vi "Welcome window.vi"(11 "error in (no error)":errorcluster) -> (8 "OK":bool, 10 "Quick start":bool, 15 "error out":errorcluster)   [LabVIEW 2011]
doc: "Welcome screen, with basic options"
uses:
  Tool/Tool selectro.ctl
  Tool/Stroker selectro.ctl
  Tool/Driller selectro.ctl
  Tool/Tractor selectro.ctl
  Project control/Project infor with project path.ctl
  Project control/Project in icluster.ctl
  Job setup/Job and site cluster.ctl
  emi cndiates/List of all contrys(combo box).ctl
  Job setup/Tool registration ID.ctl
  Project control/Run Information.ctl
  Tool/List of tools.ctl
  <vilib>/Utility/libraryn.llb/Check if File or Folder Exists.vi
  emi Lib/Basic/0 - General/App/Version/Private/_emi_Version Holder.vi
  <vilib>/Platform/browser.llb/Open URL in Default Browser (path).vi
  <vilib>/Platform/browser.llb/Open URL in Default Browser (string).vi
panel:
  in  "Tool selector":T1
  out "Project name":string
  in  "Quick start":bool
  in  "Sequenze":bool
  out "User name":string="TEST"
  in  "Change User":bool
  in  "Tool Builder":bool
  in  "IO Setup":bool
  in  "Data Sheets":bool
  in  "Promo":bool
  out "Version Full":string="Version"
  in  "Web Qinterra":bool
  in  "Web Mar-In":bool
  in  "Help":bool
  in  "Cancel":bool
  in  "OK btn":bool
  # "Beagle"
  # "Welcome"
  # "Please select operation mode to the right, then press Continue. \nFor more information press F1"
  # "Current project:"
  # "Tab header s can be changed as wanted\n\nCustom can be used for completly ccutom behavior,\nmust then highjack  an other hidden page, for settings"
  # "Add custom behavior taht cvan not be replicated by a simple cluster with valisdity checking"
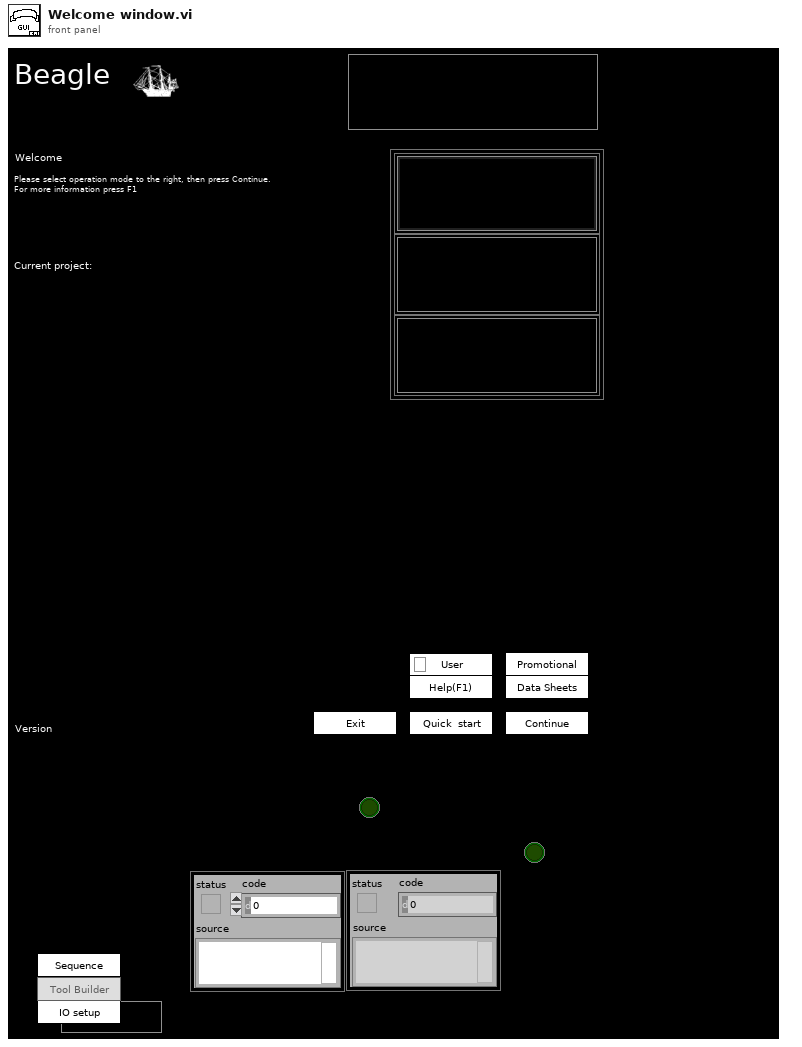
[diagram p1: front panel]
types:
  T1 = typedef "Tool selectro.ctl" = enum32{"Radio Selection 1", "Radio Selection 2", "Radio Selection 3"}
  T2 = enum32{"Invalid", "Default", "Floating", "Floating/Auto-Hide", "Modal"}
  T3 = enum16{"GET", "SET", "Get from Ini", "Put in Ini"}
  T4 = typedef "User Indikator.ctl" = cluster{"User Name":string, "Super User":T5}
  T5 = typedef "Super User bool indikator.ctl" = bool
  T6 = typedef "Options  All pages and custom.ctl" = cluster{"P 1 (App)":T7, "P 2":T8, "P 3":T9, "P 4":T12, "P 5":T17, "P 6 (Err)":T18, "P 7 (Expert)":T19, "P 8 (Depth)":T21, "C 1":T22, "C 2":T23}
  T7 = typedef "Options Page 1 (App).ctl" = cluster{"Result files":path, "PCP Interface":string, "Tractor/Stroker Interface":string, "Tractor Interface":string, "Modem Status Interface":string, "Audible Alarm":bool, "Force alarm on Technical":bool, "Force alarm on HH":bool, "Force alarm on LL":bool, "Force alarm on H":bool, "Force alarm on L":bool}
  T8 = typedef "Options Page 2.ctl" = cluster{"Solenoid & Relay latching time":u16, "Tractor relay 1":dbl, "Tractor relay 2":dbl, "Tractor Solenoid limit":dbl}
  T9 = typedef "Options Page 3.ctl" = cluster{"Min resistance":dbl, "Max resistance":dbl, "Head voltage range":T10, "Max voltage jump":dbl, "Maximum resistance change":dbl, "Start Telemetry Voltage":dbl, "Start Telemetry Timeout":dbl, "Start Motor Voltage":dbl, "Stop Motor Voltage":dbl, "Pass Mode Warning Voltage":dbl, "Relay Switch Voltage":dbl, "Relay Status Loss Voltage":dbl, "Samples to average":i32, "PSU type DO NOT USE":T11, "Magna OVP":dbl, "Magna Current Limit":dbl}
  T10 = typedef "PCP type List.ctl" = enum16{"0 - 350V", "0 - 450V", "0 - 600V"}
  T11 = typedef "PSU Type.ctl" = enum16{"Unipower", "Magna 8.3A", "Magna 12A", "None"}
  T12 = typedef "Options Page 4.ctl" = cluster{"Solenoid & Relay latching time":u16, "Stroker relay 1":dbl, "Stroker Relay 2":dbl, "Stroker Solenoid limit":dbl, "Force det.":T13, "Stroke force lim.":dbl, "Anchor Enabled Pressure":dbl, "Tacometer puls":dbl, "Default anchor behavior":T14, "Default stroker behavior":T15, "Default stroker force limit (tonne)":dbl, "Slips Size":T16}
  T13 = typedef "Stroke force selector.ctl" = enum16{"Stroke in = node 1", "Strok out = node 1"}
  T14 = typedef "Default anchor behavior.ctl" = enum16{"Do nothing", "Set Anchor", "Release Anchor"}
  T15 = typedef "Default stroker behavior.ctl" = enum16{"Do nothing", "Stop", "Go Out", "Go In"}
  T16 = typedef "Slips Type Radio.ctl" = enum32{"No Selection", "338 MRS", "3,9 MRS"}
  T17 = typedef "Options Page 5.ctl" = cluster{"Solenoid & Relay latching time":u16, "Driller relay 1":dbl, "Driller Relay 2":dbl, "Driller  Solenoid limit":dbl}
  T18 = typedef "Options Page 6 (Err).ctl" = cluster{"Error and event files":path}
  T19 = typedef "Options Page 7 (Expert).ctl" = cluster{"Show Debug":bool, "Log debug messages":bool, "Additional debug messages":bool, "Start Beagle with Simulator data":bool, "Workshop mode":bool, "Modem baud":u16, "enumCANCOM":bool, "Modem sim":T20, "Telemetry Timeout Disable":i32, "Buffer size":i32, "Upd regular data":bool, "Cable comp":cluster{"VMOD1 Voltage(V)":dbl, "VMOD2 Voltage(V)":dbl}}
  T20 = typedef "Modem simulation setup.ctl" = cluster{"Modem dealay sim":bool, "Sim baud Tx":u16, "Bit Error fraction Tx":dbl, "Sim baud Rx":u16, "Bit Error fraction Rx":dbl}
  T21 = typedef "Options Page 8 (Depth).ctl" = cluster{"Winch Spool Circumference":dbl, "Winch Pulses per Revolution":dbl, "Current Depth":dbl}
  T22 = typedef "Options Custom 1.ctl" = cluster{"Depth Updated":bool, "Depth Offset":dbl}
  T23 = typedef "Options Custom 2.ctl" = cluster{"Placeholder":bool}
  T24 = typedef "Project infor with project path.ctl" = cluster{"Project path":path, "data":T25, "Comment":string}
  T25 = typedef "Project in icluster.ctl" = cluster{"Job and Site":T26, "Tool":T28, "Run Information":T29}
  T26 = typedef "Job and site cluster.ctl" = cluster{"Project Number":string, "Client Company":string, "Country":T27, "Field":string, "Rig":string, "Well":string}
  T27 = typedef "List of all contrys(combo box).ctl" = string
  T28 = typedef "Tool registration ID.ctl" = cluster{"Tractor type":string, "Tool":string, "Serial #":string}
  T29 = typedef "Run Information.ctl" = cluster{"Active Run":bool, "String Check Rec":bool, "Run Number":i32, "Time of File Start":string}
  T30 = enum8{"Enabled", "Disabled", "Disabled and Grayed Out"}
  T31 = typedef "emi_Version Info.ctl" = cluster{"Name":string, "Major":i16, "Minor":i16, "Fix":i16, "Build":i32, "Type":enum16{"Alfa", "Beta", "Stable"}, "Dev":bool, "Version Name":string, "Date":timestamp}
  T32 = typedef "List of tools.ctl" = enum16{"Stroker", "Driller", "Tractor"}
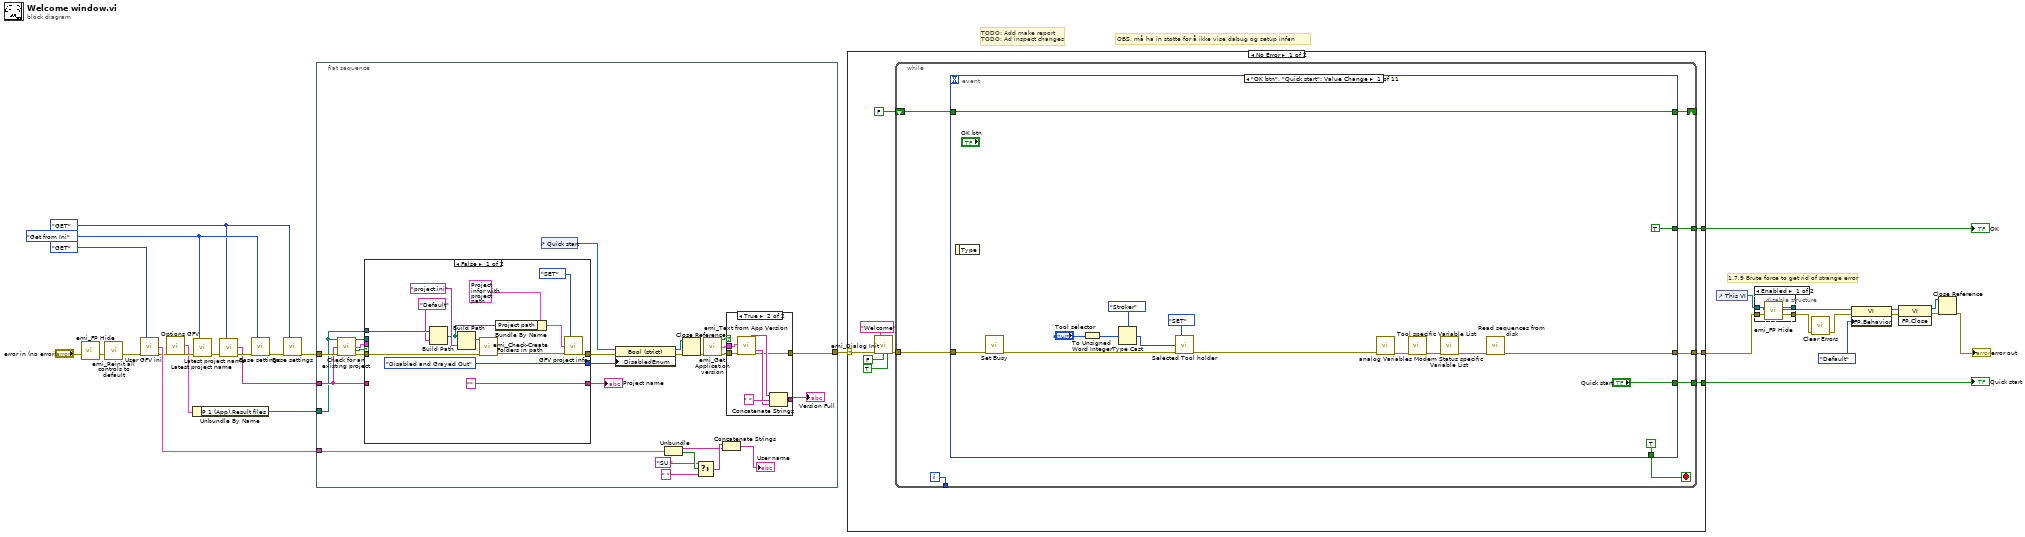
[diagram p0: block diagram]
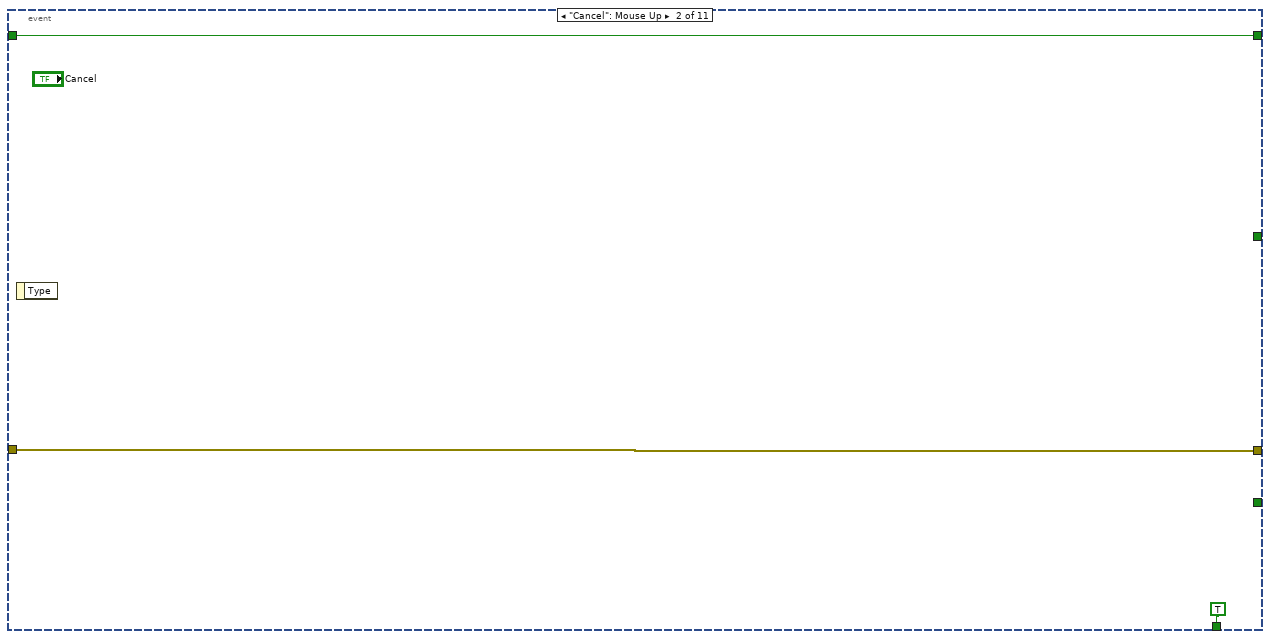
[diagram p3: hidden frame]
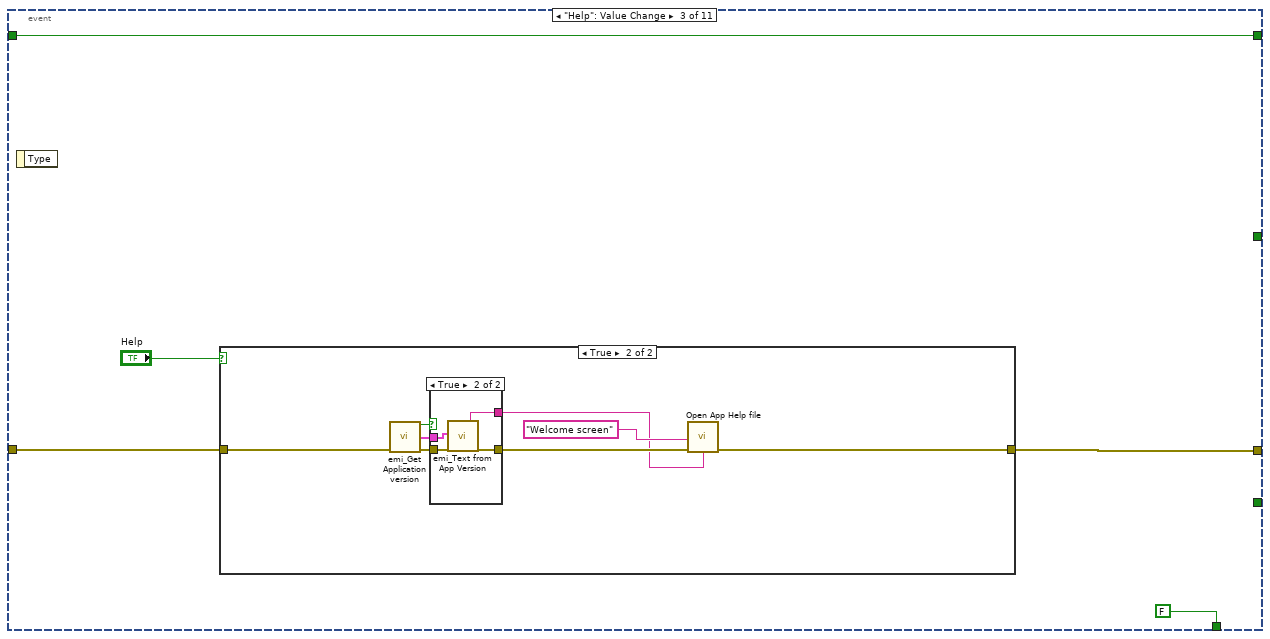
[diagram p4: hidden frame]
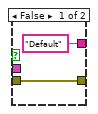
[diagram p6: hidden frame]
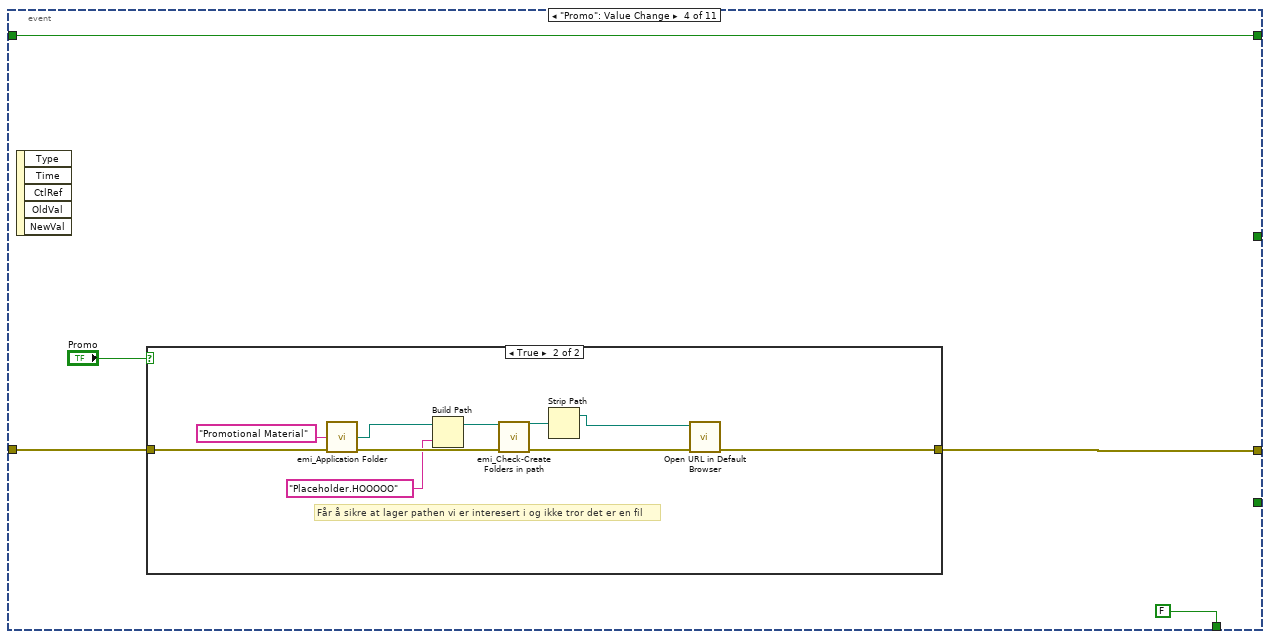
[diagram p7: hidden frame]
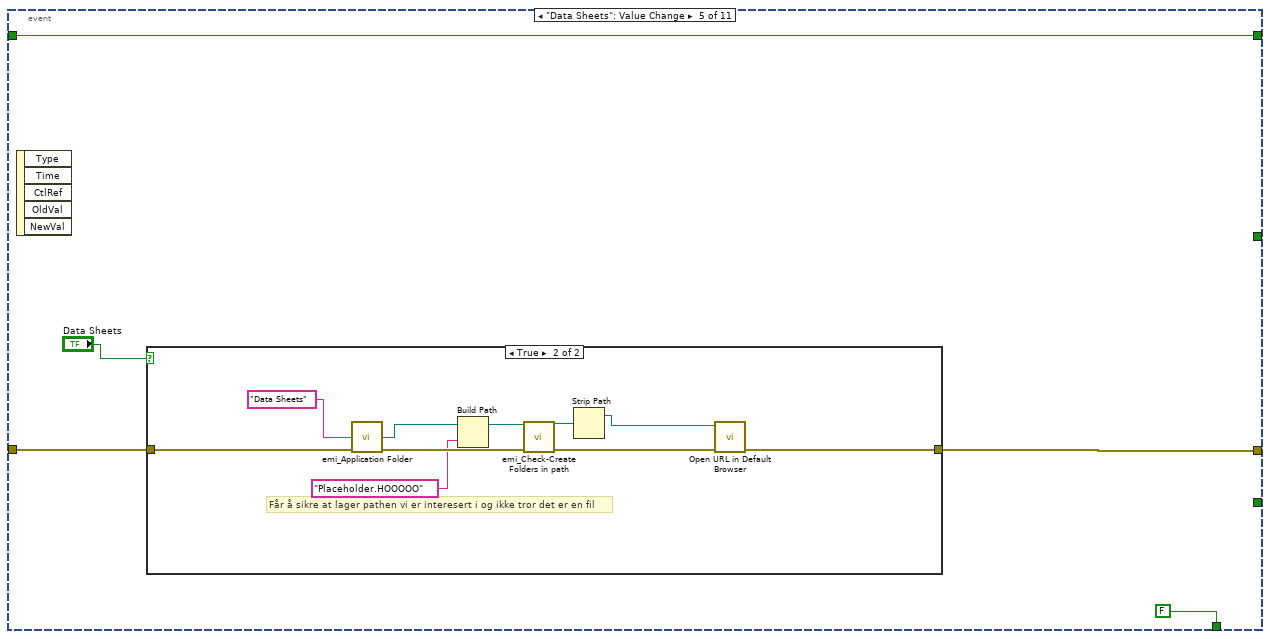
[diagram p9: hidden frame]
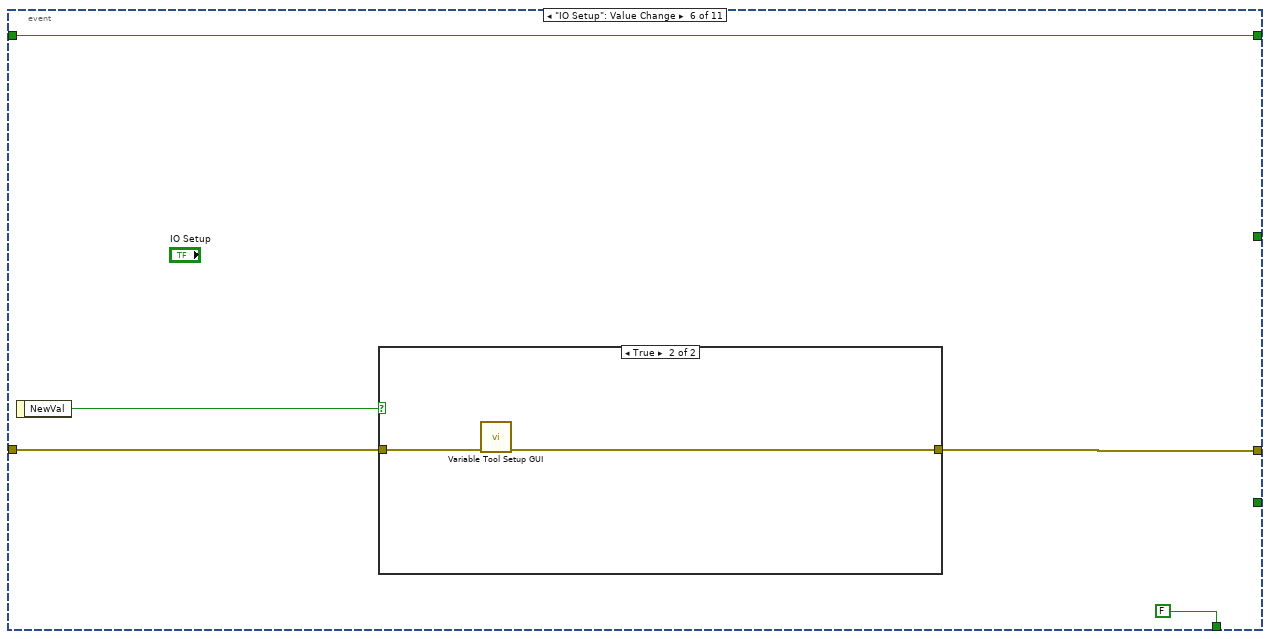
[diagram p11: hidden frame]
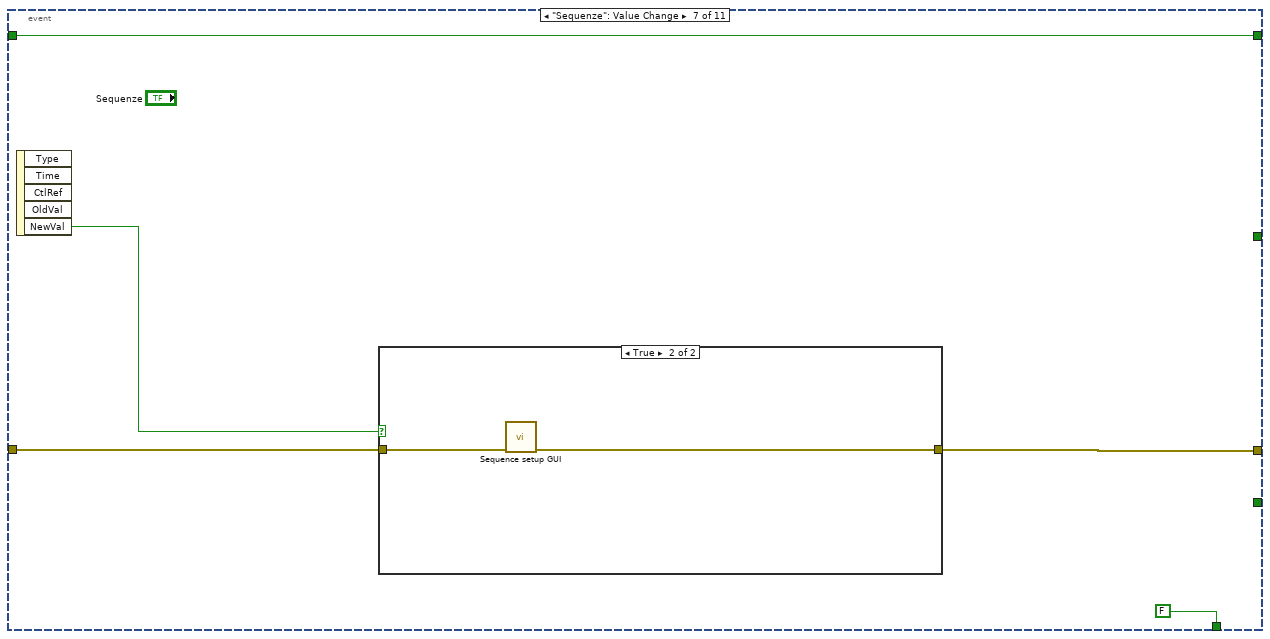
[diagram p13: hidden frame]
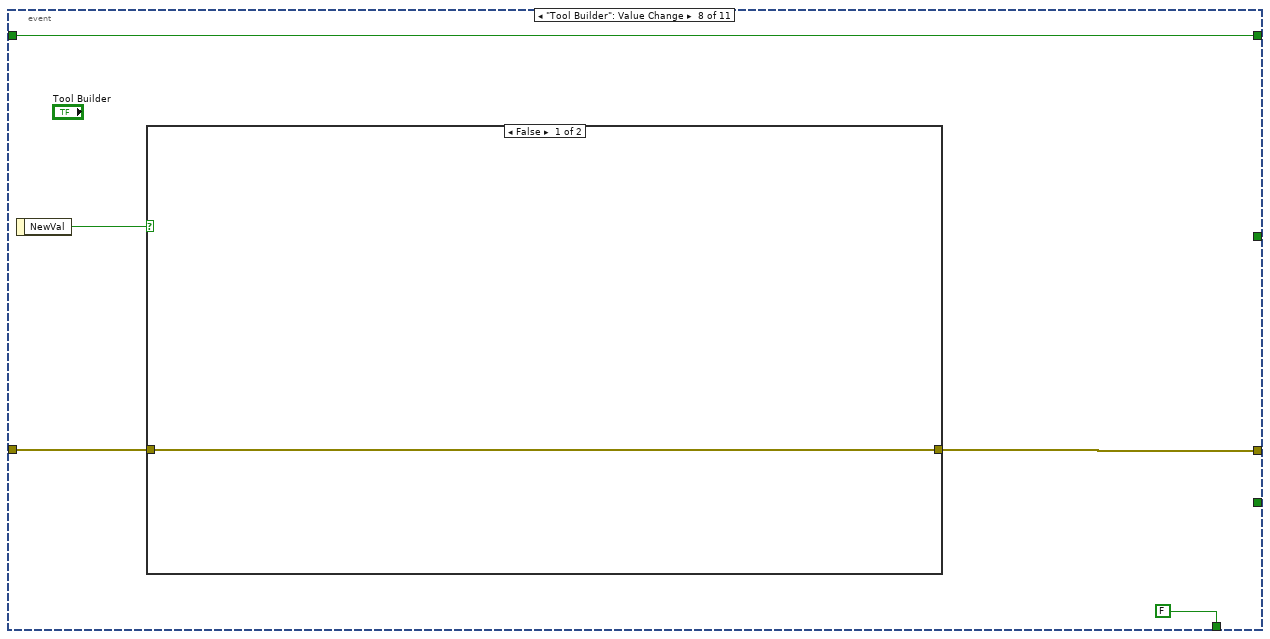
[diagram p15: hidden frame]
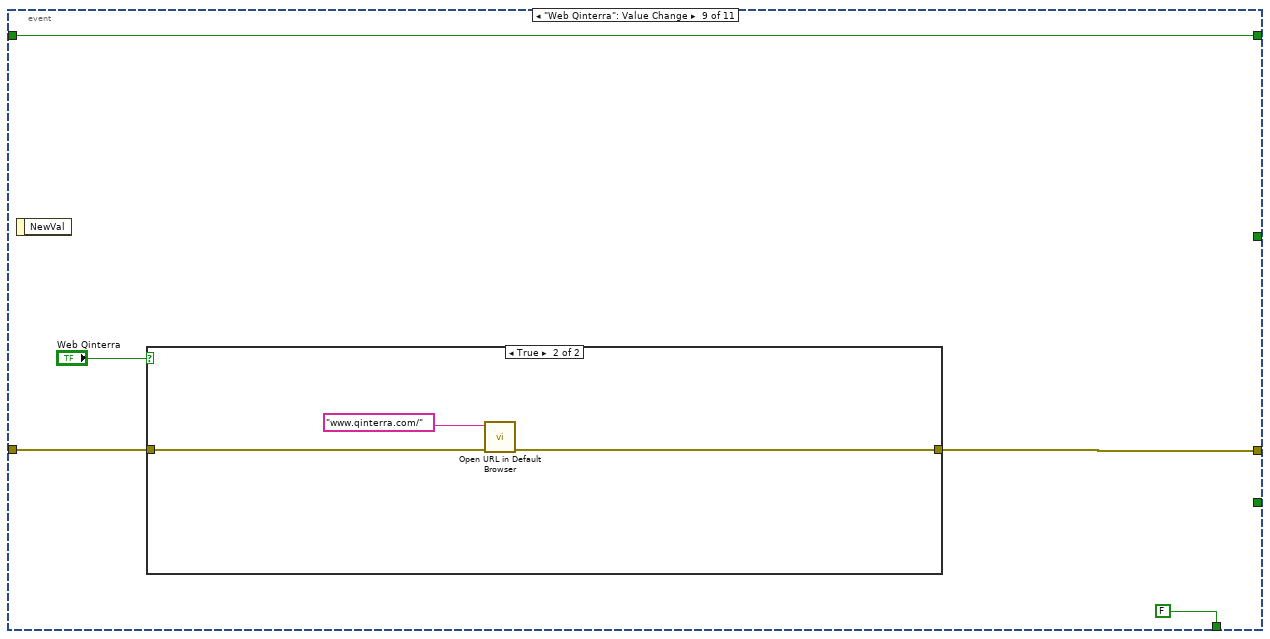
[diagram p17: hidden frame]
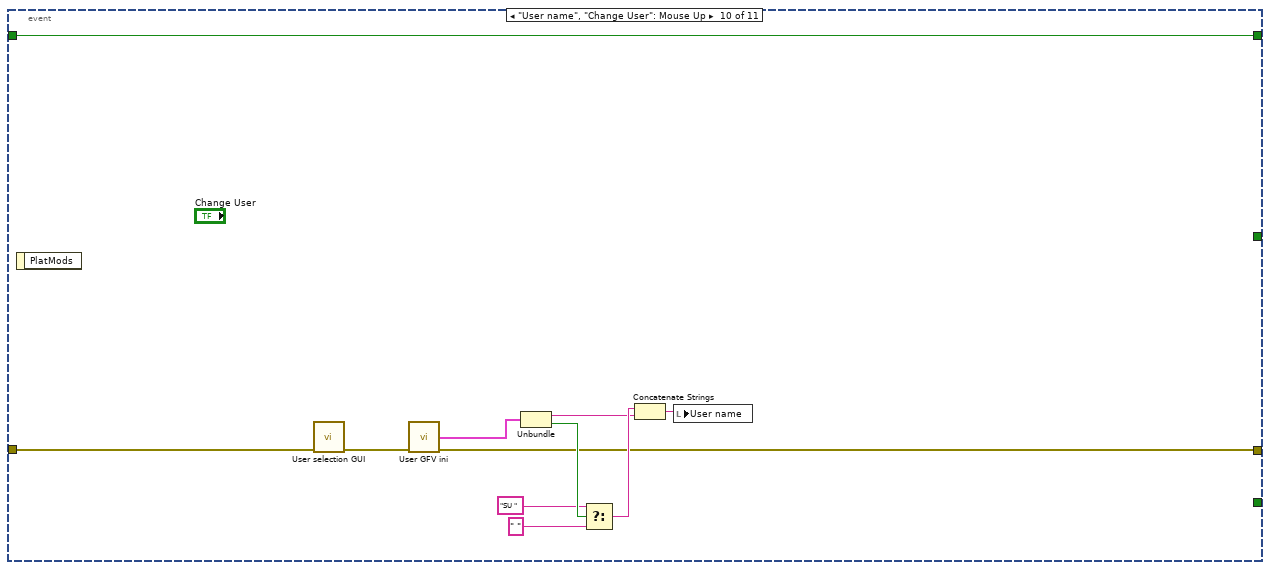
[diagram p19: hidden frame]
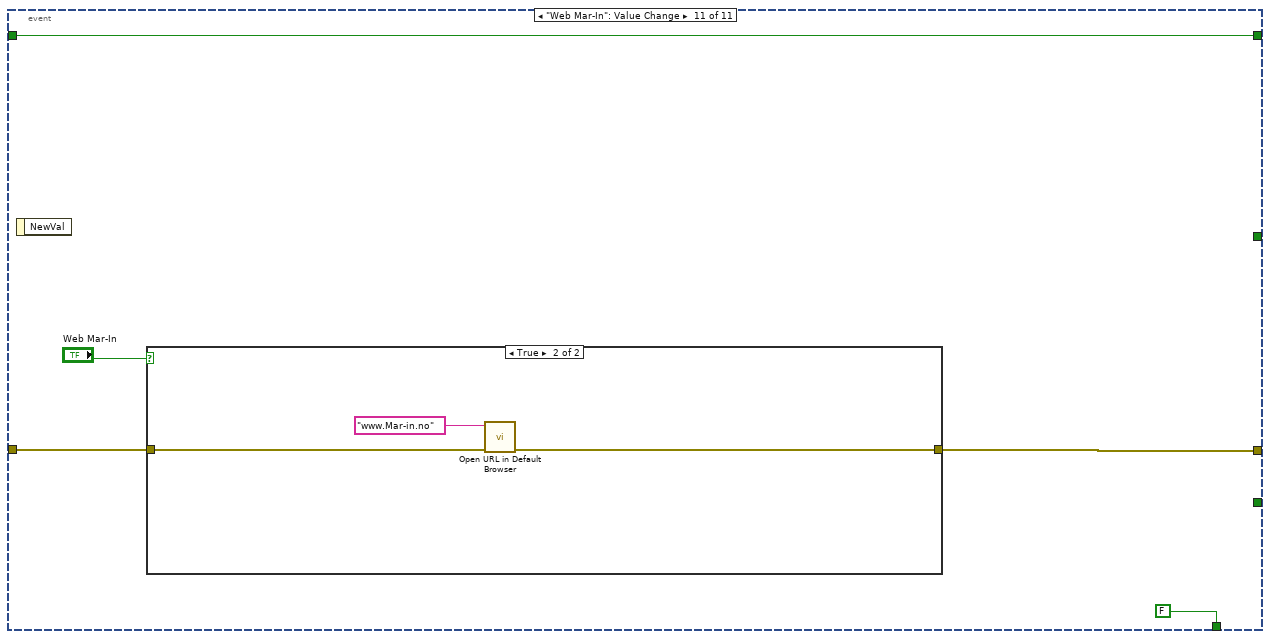
[diagram p20: hidden frame]
diagram:
  w16 = T3."GET" ("Action(GET)")
  w17 = T3."Get from Ini" ("Action(GET)")
  # "1.7.9 Brute force to get rid of strange error"
  # "OBS, må ha in støtte for å ikke vise dabug og setup infen"
  # "TODO: Add make report\nTODO: Ad inspect changes"
  n1 = call "emi_FP Hide.vi"("error in (no error)"="error in (no error)") -> ("error out"=w26:errorcluster)  [unwired: 13 in, 1 out]
  n2 = call "emi_Reinit all controls to default.vi"("error in (no error)"=w26) -> ("error out"=w1:errorcluster)  [unwired: 13 in, 1 out]
  n3 = call "User GFV ini.vi"("Action(GET)"=T3."GET", "error in (no error)"=w1) -> ("User ID out"=w23:T4, "error out"=w14:errorcluster)  [unwired: 12 in]
  n4 = call "Options GFV.vi"("error in (no error)"=w14) -> ("Options"=w12:T6, "error out"=w13:errorcluster)  [unwired: 16 in, 1 out]
  n5 = Unbundle By Name(w12) -> ("P 1 (App).Result files"=w11:path)
  n6 = call "Latest project name.vi"("Action(GET)"=w17, "error in (no error)"=w13) -> ("error out"=w19:errorcluster)  [unwired: 12 in, 1 out]
  n7 = call "Latest project name.vi"("Action(GET)"=w16, "error in (no error)"=w19) -> ("Project name out"=w15:string, "error out"=w18:errorcluster)  [unwired: 12 in]
  n8 = call "Base settings.vi"("Action(GET)"=w17, "error in (no error)"=w18) -> ("error out"=w22:errorcluster)  [unwired: 12 in, 1 out]
  n9 = call "Base settings.vi"("Action(GET)"=w16, "error in (no error)"=w22) -> ("error out"=w21:errorcluster)  [unwired: 12 in, 1 out]
  n10 = flat-sequence {
    tunnel: [w52] -> w25
    tunnel: w21 -> [w45]
    tunnel: w23 -> [w31]
    tunnel: w15 -> [w42]
    tunnel: w11 -> [w32]
    frame #0 {
      n11 = call "Check for an existing project.vi"("Base folder"=w32, "Project name"=w42, "error in"=w45) -> ("Project folder"=w34:path, "data"=w33:T25, "Project exists"=w43:bool, "error out"=w44:errorcluster)  [unwired: 5 in, 4 out]
      n12 = case shown="False" w43 {
        tunnel: [w60 w74] -> w39
        tunnel: w44 -> [w64 w75]
        tunnel: w42 -> [_ w71]
        tunnel: ["" ("f") w71] -> w41
        tunnel: [T30."Disabled and Grayed Out" ("Disabled") T30."Enabled" ("Disabled")] -> w35
        tunnel: w34 -> [_ w76]
        tunnel: w33 -> [_ w70]
        tunnel: w32 -> [w67 _]
        frame False {
          n13 = Build Path(base path=w67, name or relative path="Default") -> (appended path=w57:path)
          n14 = Build Path(base path=w57, name or relative path="project.ini") -> (appended path=w63:path)
          n15 = call "emi_Check-Create Folders in path.vi"("Path including file"=w63, "error in (no error)"=w64) -> ("error out"=w59:errorcluster)  [unwired: 11 in, 2 out]
          n16 = Bundle By Name(cluster=T24 {"Project path"=path "", "data"={"Job and Site"={"Project Number"="Default", "Client Company"="", "Country"="", "Field"="", "Rig"="", "Well"=""}, "Tool"={"Tractor type"="", "Tool"="", "Serial #"=""}, "Run Information"={"Active Run"=FALSE, "String Check Rec"=FALSE, "Run Number"=0, "Time of File Start"=""}}, "Comment"=""} ("Project info"), "Project path"=w57) -> (w61:T24)
          n17 = call "GFV project info.vi"("Action(GET)"=enum16{"GET", "SET"}."SET", "Project info in"=w61, "error in (no error)"=w59) -> ("error out"=w60:errorcluster)  [unwired: 11 in, 1 out]
        }
        frame True {
          n18 = Bundle(cluster=T24 {"Project path"=path "", "data"={"Job and Site"={"Project Number"="", "Client Company"="", "Country"="", "Field"="", "Rig"="", "Well"=""}, "Tool"={"Tractor type"="", "Tool"="", "Serial #"=""}, "Run Information"={"Active Run"=FALSE, "String Check Rec"=FALSE, "Run Number"=0, "Time of File Start"=""}}, "Comment"=""} ("Project info"), "Project path"=w76, "data"=w70) -> (w72:T24)  [unwired: 1 in]
          n19 = call "GFV project info.vi"("Action(GET)"=enum16{"GET", "SET"}."SET", "Project info in"=w72, "error in (no error)"=w75) -> ("error out"=w74:errorcluster)  [unwired: 11 in, 1 out]
        }
      }
      "Project name" <- w41
      n20 = control-ref of="Quick start"() -> (w40:refnum<vi>)
      n21 = property class="Bool (strict)"(reference=w40, error in=w39, "DisabledEnum"=w35) -> (reference out=w36:refnum<vi>, error out=w37:errorcluster)
      n22 = Unbundle(w31) -> ("User Name"=w47:string, "Super User"=w51:T5)
      n23 = Close Reference(reference=w36, error in (no error)=w37) -> (error out=w38:errorcluster)
      n24 = Select(t="SU " ("User Name"), s=w51, f=" " ("User Name")) -> (s? t:f=w48:string)
      n25 = call "emi_Get Application version.vi"("error in (no error)"=w38) -> ("Version has been set"=w56:bool, "Version Info out"=w55:T31, "error out"=w54:errorcluster)  [unwired: 12 in]
      n26 = Concatenate Strings(w48, w47) -> (→"User name":string)
      n27 = case shown="True" w56 {
        tunnel: ["" w87] -> w53
        tunnel: w54 -> [w79 w85]
        tunnel: w55 -> [_ w84]
        tunnel: [w79 w81] -> w52
        frame False {
        }
        frame True {
          n28 = call "emi_Text from App Version.vi"("Version Info"=w84, "error in (no error)"=w85) -> ("Name"=w83:string, "Full version"=w82:string, "error out"=w81:errorcluster)  [unwired: 8 in, 7 out]
          n29 = Concatenate Strings(w83, " " ("string"), w82) -> (w87:string)
        }
      }
      "Version Full" <- w53
    }
  }
  n30 = case shown="No Error" w25 {
    selector: w25 -> [w91 w233]
    tunnel: [w96 FALSE] -> w29
    tunnel: [w95 w233] -> w28
    tunnel: [w88 _] -> w20
    frame No Error {
      n31 = call "emi_Dialog Init.vi"("Header String(\"\")"="Welcome" ("Header String(\"\")"), "error in"=w91, "Set BG Color(T)"=FALSE, "Modal(T)"=TRUE) -> ("error out"=w94:errorcluster)  [unwired: 11 in]
      n32 = while {
        tunnel: [w104] -> _
        tunnel: w94 -> [w102]
        tunnel: [w101] -> w95
        tunnel: [w100] -> w96
        shift-right: [w98] -> _
        shift-left: FALSE -> [w99]
        tunnel: [w97] -> w88
        i -> [w104]
        stop <- w103 stop-if-true
        n33 = event shown="[0] \"OK btn\", \"Quick start\": Value Change" {
          selector: _ -> [_ _ _ _ _ _ _ _ _ _ _]
          dyn-events: _ -> [_ _ _ _ _ _ _ _ _ _ _]
          timeout: _ -> [_ _ _ _ _ _ _ _ _ _ _]
          tunnel: [TRUE TRUE FALSE FALSE FALSE FALSE FALSE FALSE FALSE _ FALSE] -> w103
          tunnel: w102 -> [w117 w122 w126 w146 w162 w178 w186 w194 w201 w212 w221]
          tunnel: [w115 w122 w127 w147 w163 w179 w187 w195 w202 w208 w222] -> w101
          tunnel: [TRUE _ _ _ _ _ _ _ _ _ _] -> w100
          tunnel: w99 -> [w119 w121 w124 w145 w161 w177 w185 w193 w200 w218 w220]
          tunnel: [w119 w121 w124 w145 w161 w177 w185 w193 w200 w218 w220] -> w98
          tunnel: ["Quick start" _ _ _ _ _ _ _ _ _ _] -> w97
          event "OK btn", "Quick start": Value Change {
            n34 = event-data() -> ()  [unwired: 1 in, 1 out]
            n35 = call <vilib>:"Set Busy.vi"("error in (no error)"=w117) -> ("error out"=w113:errorcluster)  [unwired: 9 in, 1 out]
            n36 = To Unsigned Word Integer(number="Tool selector") -> (unsigned 16bit integer=w111:u16)
            n37 = Type Cast(type=List_of_tools."Stroker" ("Tool in"), x=w111) -> (*(type *) &x=w109:T32)
            n38 = call "Selected Tool holder.vi"("Action(GET)"=enum16{"GET", "SET"}."SET", "Tool in"=w109, "error in (no error)"=w113) -> ("error out"=w107:errorcluster)  [unwired: 11 in, 1 out]
            n39 = call "analog Variables.vi"("error in (no error)"=w107) -> ("error out"=w108:errorcluster)  [unwired: 14 in]
            n40 = call "Tool specific Variable List.vi"("error in (no error)"=w108) -> ("error out"=w106:errorcluster)  [unwired: 14 in]
            n41 = call "Modem Status specific Variable List.vi"("error in (no error)"=w106) -> ("error out"=w105:errorcluster)  [unwired: 14 in]
            n42 = call "Read sequences from disk.vi"("error in (no error)"=w105) -> ("error out"=w115:errorcluster)  [unwired: 14 in]
          }
          event "Cancel": Mouse Up {
            n43 = event-data() -> ()  [unwired: 1 in, 1 out]
          }
          event "Help": Value Change {
            n44 = event-data() -> ()  [unwired: 1 in, 1 out]
            n45 = case shown="True" "Help" {
              tunnel: [w129 w137] -> w127
              tunnel: w126 -> [w129 w131]
              frame False {
              }
              frame True {
                n46 = call "emi_Get Application version.vi"("error in (no error)"=w131) -> ("Version has been set"=w134:bool, "Version Info out"=w133:T31, "error out"=w132:errorcluster)  [unwired: 12 in]
                n47 = case shown="True" w134 {
                  tunnel: w132 -> [w139 w143]
                  tunnel: w133 -> [_ w142]
                  tunnel: [w139 w141] -> w136
                  tunnel: ["Default" w140] -> w130
                  frame False {
                  }
                  frame True {
                    n48 = call "emi_Text from App Version.vi"("Version Info"=w142, "error in (no error)"=w143) -> ("Name"=w140:string, "error out"=w141:errorcluster)  [unwired: 8 in, 8 out]
                  }
                }
                n49 = call "Open App Help file.vi"("Help Tag (\"\")"="Welcome screen" ("Help Tag (\"\")"), "error In"=w136, "file name(\"App\".chm)"=w130) -> ("error out"=w137:errorcluster)  [unwired: 12 in]
              }
            }
          }
          event "Promo": Value Change {
            n50 = event-data() -> ()  [unwired: 1 in, 5 out]
            n51 = case shown="True" "Promo" {
              tunnel: [w149 w155] -> w147
              tunnel: w146 -> [w149 w158]
              frame False {
              }
              frame True {
                # "Får å sikre at lager pathen vi er interesert i og ikke tror det er en fil"
                n52 = call "emi_Application Folder.vi"("Sub Dir name"="Promotional Material" ("Name"), "error in (no error)"=w158) -> ("Dir"=w156:path, "error out"=w157:errorcluster)  [unwired: 12 in]
                n53 = Build Path(base path=w156, name or relative path="Placeholder.HOOOOO") -> (appended path=w154:path)
                n54 = call "emi_Check-Create Folders in path.vi"("Path including file"=w154, "error in (no error)"=w157) -> ("Path out"=w152:path, "error out"=w150:errorcluster)  [unwired: 11 in, 1 out]
                n55 = Strip Path(path=w152) -> (stripped path=w151:path)  [unwired: 1 out]
                n56 = call-poly <vilib>:"Open URL in Default Browser.vi"("error in (no error)"=w150, "path"=w151) -> ("error out"=w155:errorcluster)  [unwired: 4 in, 1 out]
              }
            }
          }
          event "Data Sheets": Value Change {
            n57 = event-data() -> ()  [unwired: 1 in, 5 out]
            n58 = case shown="True" "Data Sheets" {
              tunnel: [w165 w166] -> w163
              tunnel: w162 -> [w165 w168]
              frame False {
              }
              frame True {
                # "Får å sikre at lager pathen vi er interesert i og ikke tror det er en fil"
                n59 = call "emi_Application Folder.vi"("Sub Dir name"="Data Sheets" ("Name"), "error in (no error)"=w168) -> ("Dir"=w174:path, "error out"=w175:errorcluster)  [unwired: 12 in]
                n60 = Build Path(base path=w174, name or relative path="Placeholder.HOOOOO") -> (appended path=w173:path)
                n61 = call "emi_Check-Create Folders in path.vi"("Path including file"=w173, "error in (no error)"=w175) -> ("Path out"=w171:path, "error out"=w169:errorcluster)  [unwired: 11 in, 1 out]
                n62 = Strip Path(path=w171) -> (stripped path=w170:path)  [unwired: 1 out]
                n63 = call-poly <vilib>:"Open URL in Default Browser.vi"("error in (no error)"=w169, "path"=w170) -> ("error out"=w166:errorcluster)  [unwired: 4 in, 1 out]
              }
            }
          }
          event "IO Setup": Value Change {
            n64 = event-data() -> ("NewVal"=w176:bool)  [unwired: 1 in]
            n65 = case shown="True" w176 {
              tunnel: [w181 w182] -> w179
              tunnel: w178 -> [w181 w183]
              frame False {
              }
              frame True {
                n66 = call "Variable Tool Setup GUI.vi"("error in (no error)"=w183) -> ("error out"=w182:errorcluster)  [unwired: 13 in, 1 out]
              }
            }
          }
          event "Sequenze": Value Change {
            n67 = event-data() -> ("NewVal"=w184:bool)  [unwired: 1 in, 4 out]
            n68 = case shown="True" w184 {
              tunnel: [w189 w190] -> w187
              tunnel: w186 -> [w189 w191]
              frame False {
              }
              frame True {
                n69 = call "Sequence setup GUI.vi"("error in (no error)"=w191) -> ("error out"=w190:errorcluster)  [unwired: 13 in, 1 out]
              }
            }
          }
          event "Tool Builder": Value Change {
            n70 = event-data() -> ("NewVal"=w192:bool)  [unwired: 1 in]
            n71 = case shown="False" w192 {
              tunnel: [w197 w198] -> w195
              tunnel: w194 -> [w197 w198]
              frame False {
              }
              frame True {
              }
            }
          }
          event "Web Qinterra": Value Change {
            n72 = event-data() -> ()  [unwired: 1 in, 1 out]
            n73 = case shown="True" "Web Qinterra" {
              tunnel: [w204 w207] -> w202
              tunnel: w201 -> [w204 w206]
              frame False {
              }
              frame True {
                n74 = call-poly <vilib>:"Open URL in Default Browser.vi"("error in (no error)"=w206, "URL"="www.qinterra.com/") -> ("error out"=w207:errorcluster)  [unwired: 4 in, 1 out]
              }
            }
          }
          event "User name", "Change User": Mouse Up {
            n75 = event-data() -> ()  [unwired: 1 in, 1 out]
            n76 = call "User selection GUI.vi"("error in (no error)"=w212) -> ("error out"=w211:errorcluster)  [unwired: 13 in, 1 out]
            n77 = call "User GFV ini.vi"("error in (no error)"=w211) -> ("User ID out"=w210:T4, "error out"=w208:errorcluster)  [unwired: 13 in]
            n78 = Unbundle(w210) -> ("User Name"=w214:string, "Super User"=w217:T5)
            n79 = Select(t="SU " ("User Name"), s=w217, f=" " ("User Name")) -> (s? t:f=w215:string)
            n80 = Concatenate Strings(w215, w214) -> (w213:string)
            n81 = local write "User name"(w213) -> ()
          }
          event "Web Mar-In": Value Change {
            n82 = event-data() -> ()  [unwired: 1 in, 1 out]
            n83 = case shown="True" "Web Mar-In" {
              tunnel: [w224 w227] -> w222
              tunnel: w221 -> [w224 w226]
              frame False {
              }
              frame True {
                n84 = call-poly <vilib>:"Open URL in Default Browser.vi"("error in (no error)"=w226, "URL"="www.Mar-in.no") -> ("error out"=w227:errorcluster)  [unwired: 4 in, 1 out]
              }
            }
          }
        }
      }
    }
    frame Error {
      n85 = Unbundle(w233) -> ("code"=w230:i32, "source"=w229:string)  [unwired: 1 out]
      n86 = Format Into String(format string="%d    %s", initial string="Welcome dialog could not be displayed due to error\n\n" ("message"), w230, w229) -> (resulting string=w231:string)  [unwired: 1 in, 1 out]
      n87 = One Button Dialog(message=w231) -> ()  [unwired: 1 in, 1 out]
    }
  }
  "OK" <- w29
  "Quick start" <- w20
  n88 = control-ref of="This VI"() -> (w2:refnum<vi>)
  n89 = disable-structure shown="Enabled" {
    disable-tunnel: w2 -> [w238 w240]
    disable-tunnel: w28 -> [w237 w239]
    disable-tunnel: [w236 w240] -> w8
    disable-tunnel: [w235 w239] -> w9
    frame Enabled {
      n90 = call "emi_FP Hide.vi"("VI Refnum(This vi)"=w238, "error in (no error)"=w237) -> ("VI Refnum"=w236:refnum<vi>, "error out"=w235:errorcluster)  [unwired: 12 in]
    }
    frame Disabled {
    }
  }
  n91 = call <vilib>:"Clear Errors.vi"("error in (no error)"=w9) -> ("error out"=w10:errorcluster)  [unwired: 6 in]
  n92 = property class="VI"(reference=w8, error in=w10, "FP.Behavior"=T2."Default" ("Front Panel Window:Behavior")) -> (reference out=w7:refnum<vi>, error out=w6:errorcluster)
  n93 = invoke class="VI" method="FP.Close"(reference=w7, error in=w6) -> (reference out=w3:refnum<vi>, error out=w4:errorcluster)  [unwired: 1 in, 1 out]
  n94 = Close Reference(reference=w3, error in (no error)=w4) -> (error out=→"error out":errorcluster)
